vi "界面UI.vi"() -> ()   [LabVIEW 2016, in "超标留样集成.lvlib" / "德润DR803L超标留样.lvlib"]
uses:
  <vilib>/Utility/miscctls.llb/LVPointTypeDef.ctl
  <vilib>/Utility/config.llb/NI_LVConfig.lvlib
  <vilib>/ptbypt/NI_PtbyPt.lvlib
panel:
  out "流程计时/s":i32
  in  "单步控制":bool
  in  "设置":bool
  out "采样器进程 2":T1(ring)
  out "单次采样量":u16
  out "留样模式":T2(ring)
  out "门状态":enum16{"门开", "门关"}(ring)
  out "报警状态":enum16{"无报警", "缺水报警"}(ring)
  out "仪器时间":timestamp format="%<%Y/%m/%d %H:%M:%S>T"
  out "当前瓶号":u16
  out "采样器状态":enum16{"停止", "运行"}(ring)
  out "采样器进程":i32(listbox)
  out "流程中":bool
  in  "停止流程":bool
  in  "启动流程":bool
  in  "修改门禁密码":bool
  in  "远程复位":bool
  in  "远程留样":bool
  out "Registers":u16[](array[numeric])
  in  "采样启动":bool
  in  "停止命令":bool
  in  "切换采样器状态":bool
  in  "时间校准":bool
  out "通讯":bool
  # "只在待机时启动有效"
  # "德润DR803L超标留样"
  # "只在待机时启动有效"
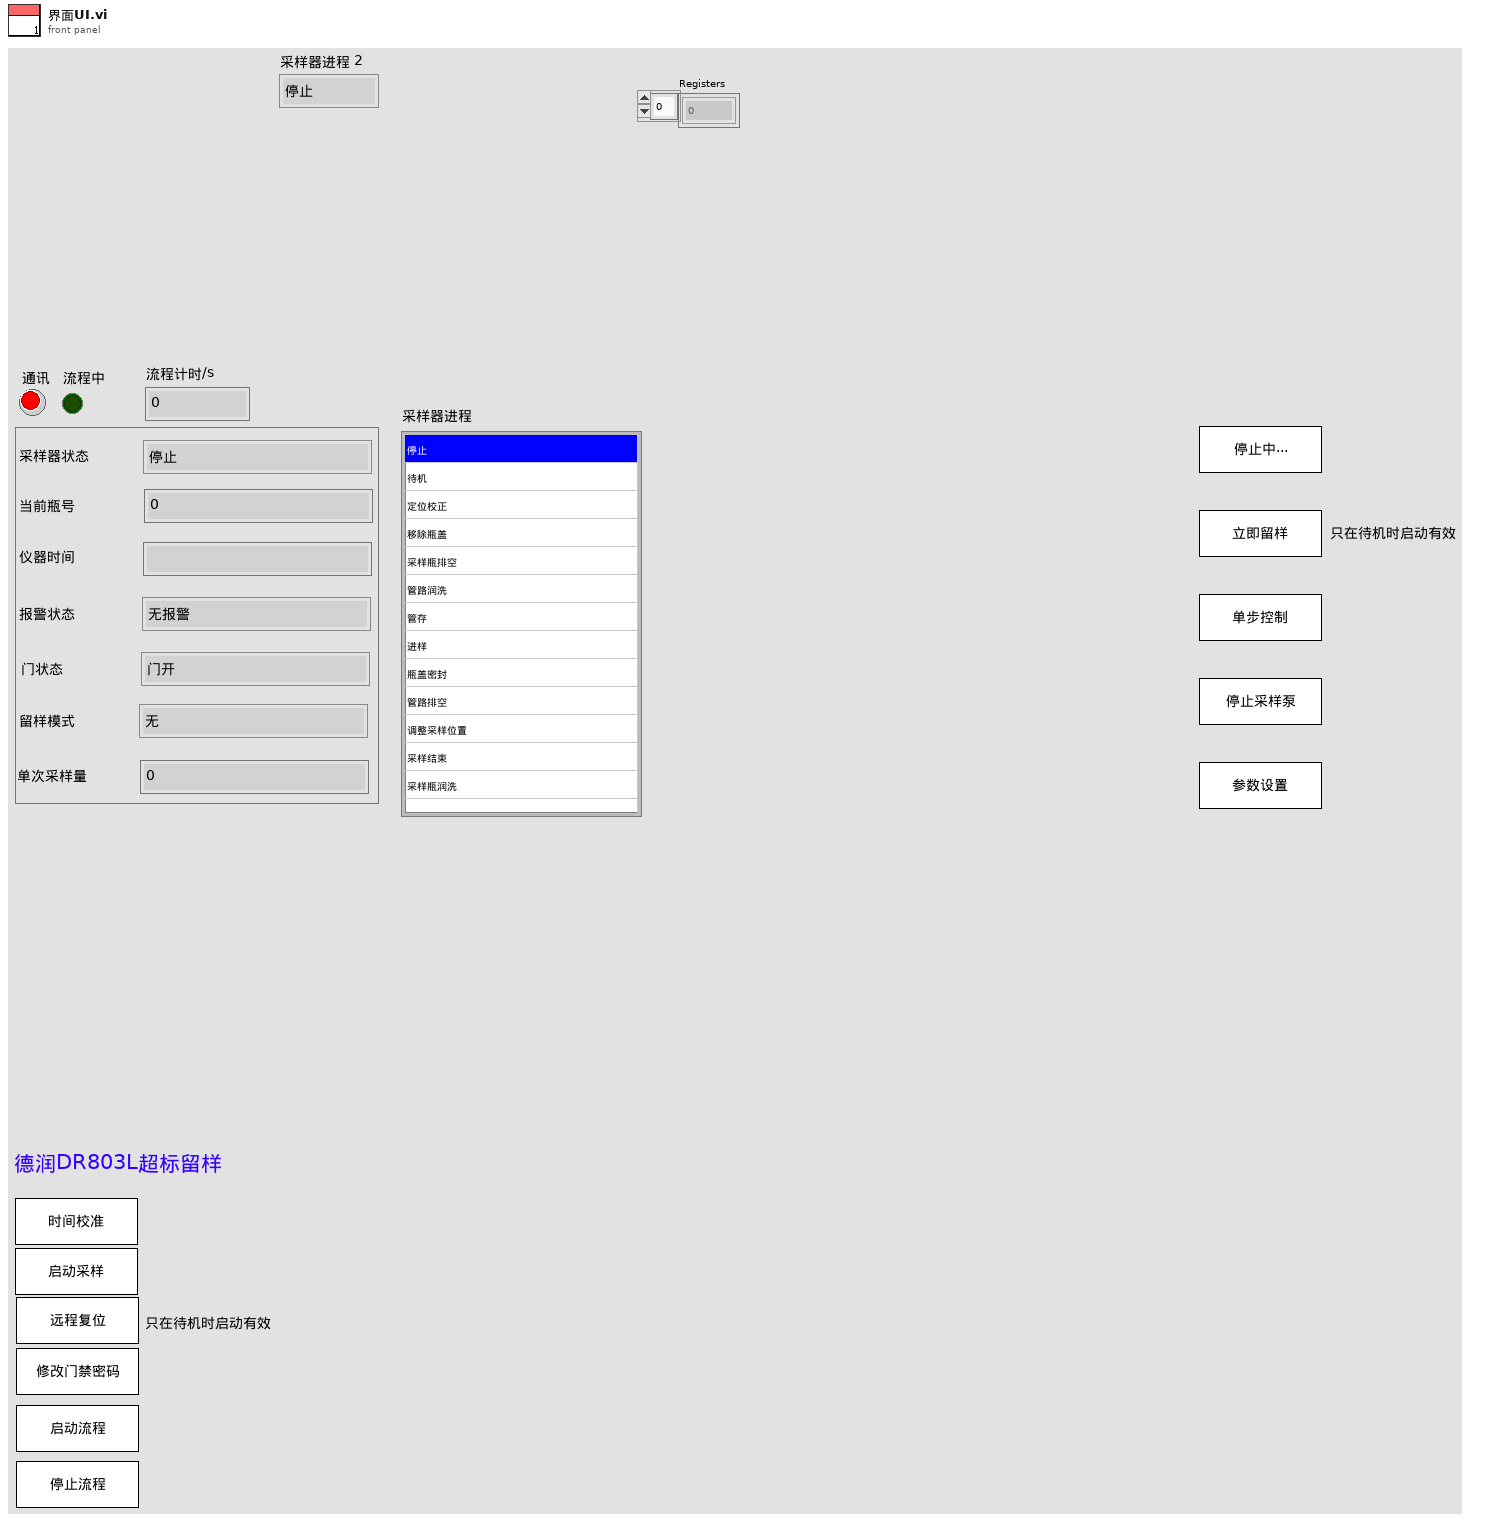
[diagram p1: front panel]
types:
  T1 = enum16{"停止", "待机", "定位校正", "移除瓶盖", "采样瓶排空", "管路润洗", "管存", "进样", "瓶盖密封", "管路排空", "调整采样位置", "采样结束", "采样瓶润洗", "瓶润洗排空"}
  T2 = enum16{"无", "定时留样", "时间等比例", "超标留样", "同步留样", "外控留样"}
  T3 = cluster{"STEP":enum16{"open", "read", "write", "write single", "close"}, "starting address":u16, "value":u16}
  T4 = typedef "LVPointTypeDef.ctl" = cluster{"Horizontal":i16, "Vertical":i16}
  T5 = typedef "NI_LVConfig.lvlib/Config Data RefNum.ctl" = refnum<k1>
  T6 = enum16{"open", "read", "write", "write single", "close"}
  T7 = typedef "LVDateTimeRec.ctl" = cluster{"秒数的小数部分":dbl, "秒":i32, "分":i32, "时":i32, "日":i32, "月":i32, "年":i32, "天数（周）":i32, "天数（年）":i32, "DST":i32}
  T8 = enum32{"Bad", "Idle", "Run top level", "Running"}
  T9 = cluster{"采样器状态":enum16{"停止", "运行"}, "当前留样瓶编号":u16, "报警状态":enum16{"无报警", "缺水报警"}, "超标信号":enum16{"无信号", "超标信号"}, "采样器进程":enum16{"停止", "待机", "定位校正", "移除瓶盖", "采样瓶排空", "管路润洗", "管存", "进样", "瓶盖密封", "管路排空", "调整采样位置", "采样结束", "采样瓶润洗", "瓶润洗排空"}, "版本号":string, "同步信号":enum16{"无信号", "同步信号"}, "外控信号":enum16{"无信号", "外控信号"}, "门状态":enum16{"门开", "门关"}, "当前瓶号":u16, "工作状态":enum16{"停止", "采样中"}, "留样模式":enum16{"无", "定时留样", "时间等比例", "超标留样", "同步留样", "外控留样"}, "立即留样":enum16{"无", "远程留样"}, "采样方式":enum16{"单采", "双重"}, "仪器时间":timestamp, "单次采样量":u16, "时间等比采样采样间隔":u16, "排空命令":u16, "远程复位":u16, "门禁密码":u16}
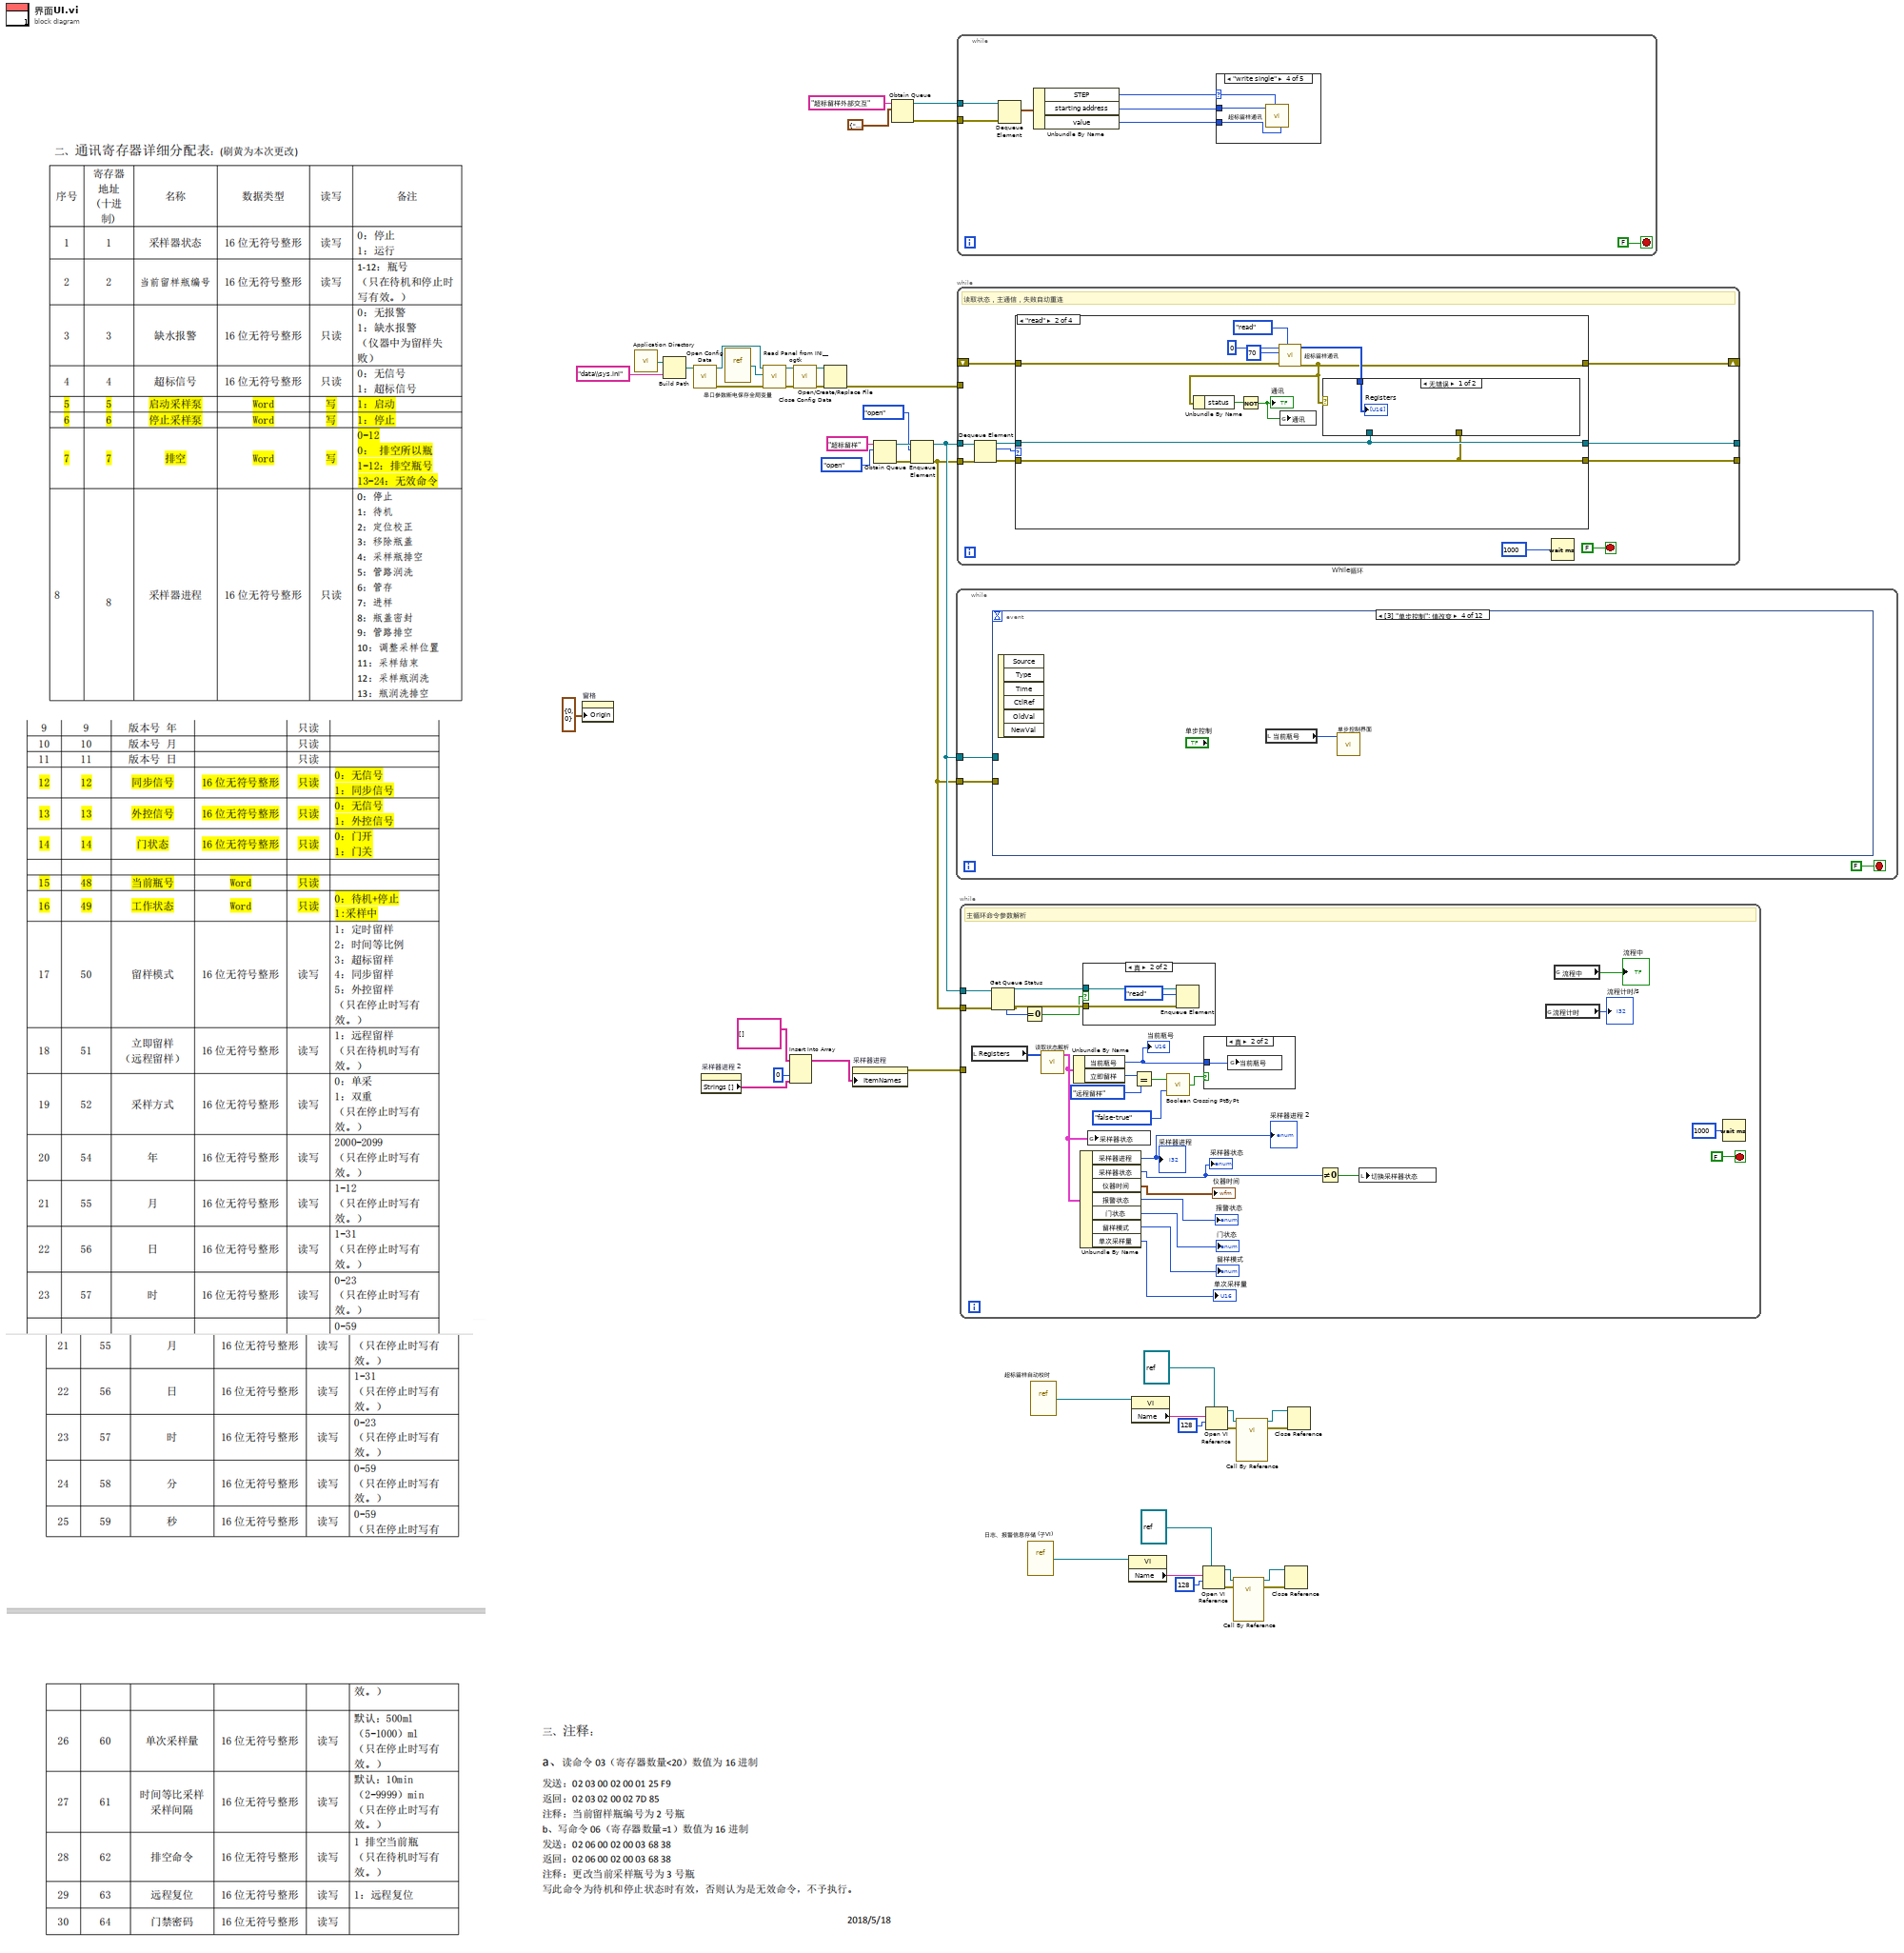
[diagram p0: block diagram]
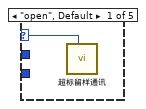
[diagram p2: hidden frame]
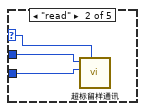
[diagram p3: hidden frame]
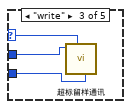
[diagram p4: hidden frame]
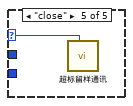
[diagram p5: hidden frame]
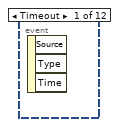
[diagram p6: hidden frame]
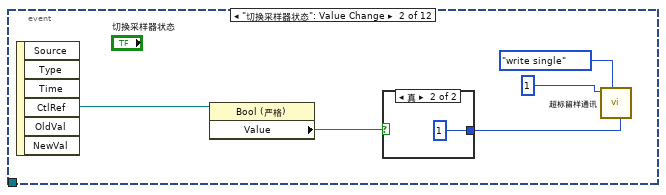
[diagram p7: hidden frame]
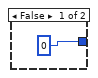
[diagram p8: hidden frame]
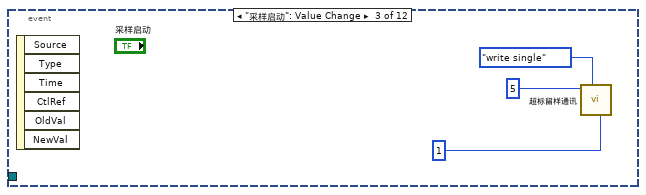
[diagram p9: hidden frame]
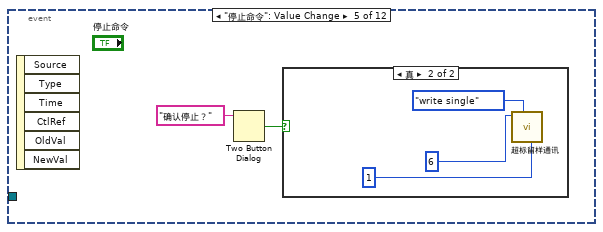
[diagram p10: hidden frame]
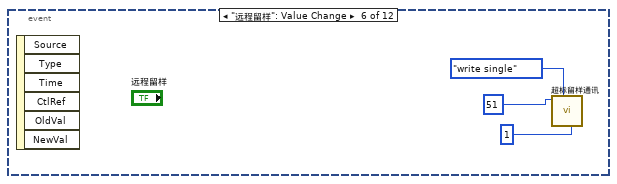
[diagram p12: hidden frame]
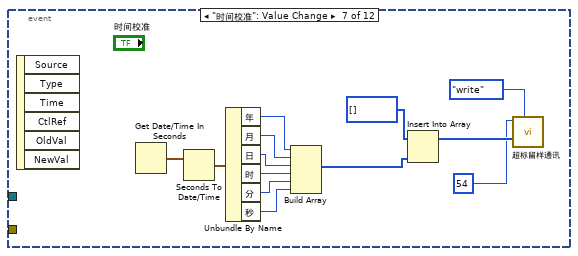
[diagram p13: hidden frame]
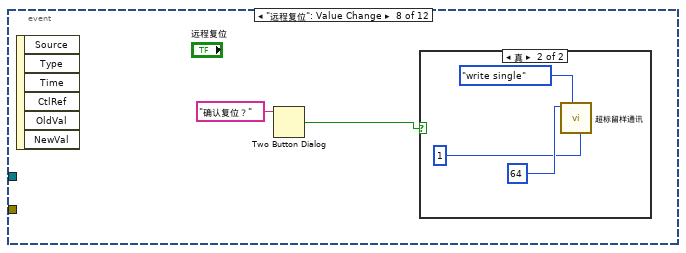
[diagram p14: hidden frame]
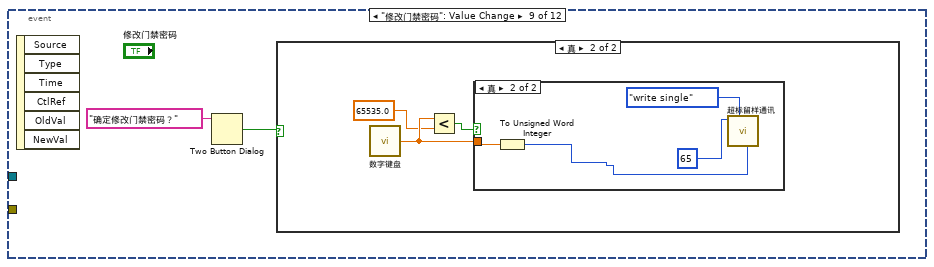
[diagram p16: hidden frame]
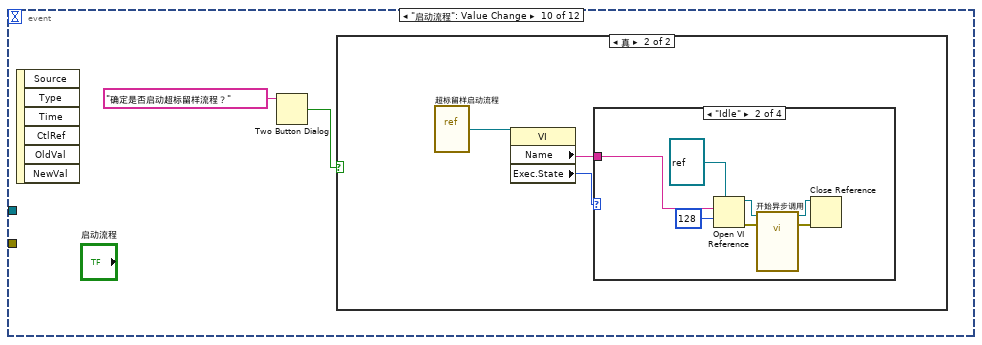
[diagram p19: hidden frame]
diagram:
  n1 = property on="窗格" class="Pane"("Origin"=T4 {"Horizontal"=0, "Vertical"=0} ("原点")) -> ()  [unwired: 2 in, 2 out]
  n2 = call <vilib>:"Application Directory.vi"() -> ("Application Directory"=w36:path)
  n3 = Build Path(base path=w36, name or relative path="data\\sys.ini" ("名称或相对路径")) -> (appended path=w34:path)
  n4 = call <vilib>:"Open Config Data.vi"("configuration file path"=w34) -> ("error out"=w30:errorcluster, "refnum"=w33:T5)  [unwired: 8 in, 1 out]
  n5 = property on="采样器进程 2" class="Enum (严格)"() -> ("Strings []"=w1:string[])  [unwired: 2 in, 2 out]
  n6 = vi-ref "串口参数断电保存全局变量.vi"() -> (w32:refnum<vi>)
  n7 = call <userlib>:"Read Panel from INI__ogtk.vi"("error in (no error)"=w30, "VI ref"=w32, "refnum"=w33) -> ("error out"=w29:errorcluster, "refnum out"=w31:T5)  [unwired: 7 in]
  n8 = Insert Into Array(array=string[][] [] ("字符串[]"), index (col)=0 ("禁用的索引 (列)"), new element=w1) -> (w3:string[][])  [unwired: 1 in]
  n9 = call <vilib>:"Close Config Data.vi"("error in (no error)"=w29, "refnum"=w31) -> ("error out"=w28:errorcluster, "file path"=w27:path)  [unwired: 8 in]
  n10 = Open/Create/Replace File(file path (use dialog)=w27, error in=w28) -> (error out=w26:errorcluster)  [unwired: 4 in, 2 out]
  n11 = property on="采样器进程" class="MCListbox (严格)"("ItemNames"=w3) -> (error out=w2:errorcluster)  [unwired: 2 in, 1 out]
  n12 = Obtain Queue(name (unnamed)="超标留样" ("名称（未命名）"), element data type=enum16{"open", "read", "write", "close"}."open") -> (queue out=w42:refnum<queue>, error out=w41:errorcluster)  [unwired: 3 in, 1 out]
  n13 = Obtain Queue(name (unnamed)="超标留样外部交互" ("名称（未命名）"), element data type=T3 {"STEP"=enum."write single", "starting address"=0, "value"=0}) -> (queue out=w23:refnum<queue>, error out=w22:errorcluster)  [unwired: 3 in, 1 out]
  n14 = Enqueue Element(queue=w42, element=enum16{"open", "read", "write", "close"}."open", error in (no error)=w41) -> (queue out=w39:refnum<queue>, error out=w38:errorcluster)  [unwired: 1 in, 1 out]
  n15 = while {
    tunnel: w39 -> [w46]
    tunnel: w38 -> [w45]
    stop <- FALSE stop-if-true
    n16 = event shown="[3] \"单步控制\": 值改变" {
      selector: _ -> [_ _ _ _ _ _ _ _ _ _ _ _]
      dyn-events: _ -> [_ _ _ _ _ _ _ _ _ _ _ _]
      timeout: _ -> [_ _ _ _ _ _ _ _ _ _ _ _]
      tunnel: w46 -> [_ _ _ _ _ _ _ _ _ _ _ _]
      tunnel: w45 -> [_ _ _ _ _ _ _ _ _ _ _ _]
      event Timeout {
        n17 = event-data() -> ()  [unwired: 1 in, 3 out]
      }
      event "切换采样器状态": Value Change {
        n18 = event-data() -> ("CtlRef"=w52:refnum<vi>)  [unwired: 1 in, 5 out]
        n19 = property class="Bool (严格)"(reference=w52) -> ("Value"=w51:bool)  [unwired: 1 in, 2 out]
        n20 = case shown="真" w51 {
          tunnel: [u16 0 ("索引") u16 1 ("索引")] -> w48
          frame False {
          }
          frame True {
          }
        }
        n21 = call "超标留样通讯.vi"("value"=w48, "STEP"=T6."write single", "starting address"=1 ("索引")) -> ()  [unwired: 6 in, 3 out]
      }
      event "采样启动": Value Change {
        n22 = event-data() -> ()  [unwired: 1 in, 6 out]
        n23 = call "超标留样通讯.vi"("value"=u16 1 ("新元素/子数组"), "STEP"=T6."write single", "starting address"=5 ("索引")) -> ()  [unwired: 6 in, 3 out]
      }
      event "单步控制": Value Change {
        n24 = event-data() -> ()  [unwired: 1 in, 6 out]
        n25 = local read "当前瓶号"() -> (w58:u16)
        n26 = call "单步控制界面.vi"("当前瓶号"=w58) -> ()  [unwired: 11 in]
      }
      event "停止命令": Value Change {
        n27 = event-data() -> ()  [unwired: 1 in, 6 out]
        n28 = Two Button Dialog(message="确认停止？" ("消息")) -> (T button?=w59:bool)  [unwired: 2 in]
        n29 = case shown="真" w59 {
          frame False {
          }
          frame True {
            n30 = call "超标留样通讯.vi"("value"=u16 1 ("新元素/子数组"), "STEP"=T6."write single", "starting address"=6 ("索引")) -> ()  [unwired: 6 in, 3 out]
          }
        }
      }
      event "远程留样": Value Change {
        n31 = event-data() -> ()  [unwired: 1 in, 6 out]
        n32 = call "超标留样通讯.vi"("value"=u16 1 ("新元素/子数组"), "STEP"=T6."write single", "starting address"=51 ("索引")) -> ()  [unwired: 6 in, 3 out]
      }
      event "时间校准": Value Change {
        n33 = event-data() -> ()  [unwired: 1 in, 6 out]
        n34 = Get Date/Time In Seconds() -> (seconds since 1Jan1904=w79:timestamp)
        n35 = Seconds To Date/Time(time stamp (now)=w79) -> (date time rec=w78:T7)  [unwired: 1 in]
        n36 = Unbundle By Name(w78) -> ("年"=w75:i32, "月"=w74:i32, "日"=w73:i32, "时"=w72:i32, "分"=w71:i32, "秒"=w70:i32)
        n37 = Build Array(w75, w74, w73, w72, w71, w70) -> (w69:i32[])
        n38 = Insert Into Array(array=u16[] [] ("values"), new element=w69) -> (w76:u16[])  [unwired: 1 in]
        n39 = call "超标留样通讯.vi"("STEP"=T6."write", "values"=w76, "starting address"=54 ("索引")) -> ()  [unwired: 6 in, 3 out]
      }
      event "远程复位": Value Change {
        n40 = event-data() -> ()  [unwired: 1 in, 6 out]
        n41 = Two Button Dialog(message="确认复位？" ("消息")) -> (T button?=w80:bool)  [unwired: 2 in]
        n42 = case shown="真" w80 {
          frame False {
          }
          frame True {
            n43 = call "超标留样通讯.vi"("value"=u16 1 ("新元素/子数组"), "STEP"=T6."write single", "starting address"=64 ("索引")) -> ()  [unwired: 6 in, 3 out]
          }
        }
      }
      event "修改门禁密码": Value Change {
        n44 = event-data() -> ()  [unwired: 1 in, 6 out]
        n45 = Two Button Dialog(message="确定修改门禁密码？" ("消息")) -> (T button?=w85:bool)  [unwired: 2 in]
        n46 = case shown="真" w85 {
          frame False {
          }
          frame True {
            n47 = call "数字键盘.vi"() -> ("NewNumber"=w89:sgl)  [unwired: 1 in]
            n48 = Less?(x=w89, y=sgl 65535.0) -> (x < y?=w87:bool)
            n49 = case shown="真" w87 {
              tunnel: w89 -> [_ w93]
              frame False {
              }
              frame True {
                n50 = To Unsigned Word Integer(number=w93) -> (unsigned 16bit integer=w90:u16)
                n51 = call "超标留样通讯.vi"("value"=w90, "STEP"=T6."write single", "starting address"=65 ("索引")) -> ()  [unwired: 6 in, 3 out]
              }
            }
          }
        }
      }
      event "启动流程": Value Change {
        n52 = event-data() -> ()  [unwired: 1 in, 6 out]
        n53 = Two Button Dialog(message="确定是否启动超标留样流程？" ("消息")) -> (T button?=w94:bool)  [unwired: 2 in]
        n54 = case shown="真" w94 {
          frame False {
          }
          frame True {
            n55 = vi-ref "超标留样启动流程.vi"() -> (w96:refnum<vi>)
            n56 = property class="VI"(reference=w96) -> ("Name"=w97:string, "Exec.State"=w98:T8)  [unwired: 1 in, 2 out]
            n57 = case shown="\"Idle\"" w98 {
              tunnel: w97 -> [_ w101 _ _]
              frame "Bad", Default {
              }
              frame "Idle" {
                n58 = Open VI Reference(type specifier VI Refnum (for type only)=refnum<vi> refnum ("类型说明符VI引用句柄（仅用于类型）"), vi path=w101, options=128 ("选项")) -> (vi reference=w105:refnum<vi>, error out=w100:errorcluster)  [unwired: 3 in]
                n59 = call-by-ref "开始异步调用"(reference=w105, error in=w100) -> (reference out=w104:refnum<vi>, error out=w99:errorcluster)  [unwired: 12 in]
                n60 = Close Reference(reference=w104, error in (no error)=w99) -> ()  [unwired: 1 out]
              }
              frame "Run top level" {
              }
              frame "Running" {
              }
            }
          }
        }
      }
      event "停止流程": Value Change {
        n61 = event-data() -> ()  [unwired: 1 in, 6 out]
        n62 = Two Button Dialog(message="确定是否停止超标留样流程并排空当前瓶？" ("消息")) -> (T button?=w106:bool)  [unwired: 2 in]
        n63 = case shown="真" w106 {
          frame False {
          }
          frame True {
            n64 = Obtain Notifier(name (unnamed)="超标留样流程" ("名称（未命名）"), notification data type=FALSE ("采样完成")) -> (notifier out=w119:refnum<notifier>, error out=w118:errorcluster)  [unwired: 2 in, 1 out]
            n65 = Send Notification(notification=TRUE ("通知"), notifier=w119, error in (no error)=w118) -> (notifier out=w116:refnum<notifier>, error out=w115:errorcluster)
            n66 = call "超标留样通讯.vi"("value"=u16 1 ("新元素/子数组"), "STEP"=T6."write single", "starting address"=6 ("索引")) -> ("error out"=w108:errorcluster)  [unwired: 6 in, 2 out]
            n67 = Release Notifier(notifier=w116, error in (no error)=w115) -> ()  [unwired: 1 in, 3 out]
            n68 = call "超标留样通讯.vi"("value"=u16 1 ("新元素/子数组"), "STEP"=T6."write single", "Error in"=w108, "starting address"=63 ("索引")) -> ()  [unwired: 5 in, 3 out]
          }
        }
      }
      event "设置": Value Change {
        n69 = event-data() -> ()  [unwired: 1 in, 6 out]
        n70 = global read "超标留样全局.vi" "采样器状态"() -> (w126:T9)
        n71 = Unbundle By Name(w126) -> ("留样模式"=w125:T2, "采样方式"=w124:enum16{"单采", "双重"}, "单次采样量"=w123:u16, "时间等比采样采样间隔"=w122:u16)
        n72 = call "参数设置对画框.vi"("时间等比采样"=w122, "单次采样量"=w123, "采样方式"=w124, "留样模式"=w125) -> ()  [unwired: 8 in]
      }
    }
  }
  n73 = while {
    tunnel: w23 -> [w132]
    tunnel: w22 -> [w131]
    stop <- FALSE stop-if-true
    n74 = Dequeue Element(queue=w132, error in (no error)=w131) -> (element=w130:T3)  [unwired: 1 in, 3 out]
    n75 = Unbundle By Name(w130) -> ("STEP"=w129:T6, "starting address"=w128:u16, "value"=w127:u16)
    n76 = case shown="\"write single\"" w129 {
      selector: w129 -> [w134 w137 w140 w143 w144]
      tunnel: w128 -> [_ w136 w139 w142 _]
      tunnel: w127 -> [_ w135 w138 w141 _]
      frame "open", Default {
        n77 = call "超标留样通讯.vi"("STEP"=w134) -> ()  [unwired: 8 in, 3 out]
      }
      frame "read" {
        n78 = call "超标留样通讯.vi"("STEP"=w137, "quantity"=w135, "starting address"=w136) -> ()  [unwired: 6 in, 3 out]
      }
      frame "write" {
        n79 = call "超标留样通讯.vi"("value"=w138, "STEP"=w140, "starting address"=w139) -> ()  [unwired: 6 in, 3 out]
      }
      frame "write single" {
        n80 = call "超标留样通讯.vi"("value"=w141, "STEP"=w143, "starting address"=w142) -> ()  [unwired: 6 in, 3 out]
      }
      frame "close" {
        n81 = call "超标留样通讯.vi"("STEP"=w144) -> ()  [unwired: 8 in, 3 out]
      }
    }
  }
  n82 = while "While循环" {
    tunnel: w39 -> [w146]
    tunnel: w38 -> [w145]
    tunnel: [w150] -> _
    tunnel: [w149] -> _
    shift-right: [w147] -> _
    shift-left: _ -> [w148]
    tunnel: w26 -> [_]
    stop <- FALSE stop-if-true
    # "读取状态，主通信，失败自动重连"
    n83 = Dequeue Element(queue=w146, error in (no error)=w145) -> (queue out=w152:refnum<queue>, element=w153:enum16{"open", "read", "write", "close"}, error out=w151:errorcluster)  [unwired: 1 in, 1 out]
    n84 = case shown="\"read\"" w153 {
      tunnel: [w161 w163 w181 w190] -> w147
      tunnel: w152 -> [w160 w166 w180 w193]
      tunnel: w151 -> [w159 w165 w179 w192]
      tunnel: [w160 w166 w180 w193] -> w150
      tunnel: [w159 w165 w179 w192] -> w149
      tunnel: w148 -> [w158 w171 w183 w194]
      frame "open", Default {
        n85 = call "超标留样通讯.vi"("STEP"=T6."open", "Error in"=w158) -> ("error out"=w161:errorcluster, "MB session in"=w157:refnum<class "MB_Master.lvclass">)  [unwired: 7 in, 1 out]
        n86 = global write "串口参数断电保存全局变量.vi" "MB session in"(w157) -> ()
      }
      frame "read" {
        n87 = call "超标留样通讯.vi"("STEP"=T6."read", "Error in"=w171, "quantity"=u16 70, "starting address"=u16 0) -> ("error out"=w163:errorcluster, "Registers"=w168:u16[])  [unwired: 5 in, 1 out]
        n88 = Unbundle By Name(w163) -> ("status"=w164:bool)
        n89 = Not(x=w164) -> (.not. x?=w162:bool)
        "通讯" <- w162
        n90 = global write "超标留样全局.vi" "通讯"(w162) -> ()
        n91 = case shown="无错误" w163 {
          tunnel: w168 -> [w172 _]
          tunnel: w166 -> [_ w177]
          tunnel: w165 -> [_ w176]
          frame No Error {
            "Registers" <- w172
          }
          frame Error {
            n92 = Enqueue Element(queue=w177, element=enum16{"open", "read", "write", "close"}."close" ("元素"), error in (no error)=w176) -> (queue out=w175:refnum<queue>, error out=w174:errorcluster)  [unwired: 1 in, 1 out]
            n93 = Enqueue Element(queue=w175, element=enum16{"open", "read", "write", "close"}."open" ("元素"), error in (no error)=w174) -> ()  [unwired: 1 in, 3 out]
          }
        }
      }
      frame "write" {
        n94 = call "超标留样通讯.vi"("STEP"=T6."write single", "Error in"=w183) -> ("error out"=w181:errorcluster)  [unwired: 7 in, 2 out]
        n95 = case shown="错误" w181 {
          tunnel: w180 -> [_ w185]
          tunnel: w179 -> [_ w184]
          frame No Error {
          }
          frame Error {
            n96 = Enqueue Element(queue=w185, element=enum16{"open", "read", "write", "close"}."close" ("元素"), error in (no error)=w184) -> (queue out=w188:refnum<queue>, error out=w187:errorcluster)  [unwired: 1 in, 1 out]
            n97 = Enqueue Element(queue=w188, element=enum16{"open", "read", "write", "close"}."open" ("元素"), error in (no error)=w187) -> ()  [unwired: 1 in, 3 out]
          }
        }
      }
      frame "close" {
        n98 = call "超标留样通讯.vi"("STEP"=T6."close", "Error in"=w194) -> ("error out"=w190:errorcluster)  [unwired: 7 in, 2 out]
      }
    }
    n99 = Wait (ms)(milliseconds to wait=u32 1000 ("等待时间（毫秒）")) -> ()  [unwired: 1 out]
  }
  n100 = while {
    tunnel: w39 -> [w218]
    tunnel: w38 -> [w217]
    tunnel: w2 -> [_]
    stop <- FALSE stop-if-true
    # "主循环命令参数解析"
    n101 = local read "Registers"() -> (w212:u16[])
    n102 = Get Queue Status(queue=w218, error in (no error)=w217) -> (queue out=w215:refnum<queue>, error out=w214:errorcluster, # elements in queue=w216:i32)  [unwired: 1 in, 5 out]
    n103 = Equal To 0?(x=w216) -> (x = 0?=w213:bool)
    n104 = call "读取状态解析.vi"("Registers"=w212) -> ("采样器状态"=w205:T9)  [unwired: 9 in, 1 out]
    n105 = Unbundle By Name(w205) -> ("当前瓶号"=w204:u16, "立即留样"=w211:enum16{"无", "远程留样"})
    "当前瓶号" <- w204
    n106 = Unbundle By Name(w205) -> ("采样器进程"=→"采样器进程" →"采样器进程 2":T1, "采样器状态"=w197:enum16{"停止", "运行"}, "仪器时间"=→"仪器时间":timestamp, "报警状态"=→"报警状态":enum16{"无报警", "缺水报警"}, "门状态"=→"门状态":enum16{"门开", "门关"}, "留样模式"=→"留样模式":T2, "单次采样量"=→"单次采样量":u16)
    "采样器状态" <- w197
    n107 = case shown="真" w213 {
      tunnel: w215 -> [_ w223]
      tunnel: w214 -> [_ w222]
      frame False {
      }
      frame True {
        n108 = Enqueue Element(queue=w223, element=enum16{"open", "read", "write", "close"}."read" ("元素"), error in (no error)=w222) -> ()  [unwired: 1 in, 3 out]
      }
    }
    n109 = global write "超标留样全局.vi" "采样器状态"(w205) -> ()
    n110 = Equal?(x=w211, y=enum16{"无", "远程留样"}."远程留样") -> (x = y?=w210:bool)
    n111 = call <vilib>:"Boolean Crossing PtByPt.vi"("direction"=enum16{"either", "false-true", "true-false"}."false-true", "input"=w210) -> ("crossing"=w208:bool)  [unwired: 1 in]
    n112 = case shown="真" w208 {
      tunnel: w204 -> [_ w221]
      frame False {
      }
      frame True {
        n113 = global write "超标留样全局.vi" "当前瓶号"(w221) -> ()
      }
    }
    n114 = Not Equal To 0?(x=w197) -> (x != 0?=w196:bool)
    n115 = local write "切换采样器状态"(w196) -> ()
    n116 = global read "串口参数断电保存全局变量.vi" "流程计时"() -> (→"流程计时/s":i32)
    n117 = global read "串口参数断电保存全局变量.vi" "流程中"() -> (→"流程中":bool)
    n118 = Wait (ms)(milliseconds to wait=u32 1000 ("等待时间（毫秒）")) -> ()  [unwired: 1 out]
  }
  n119 = vi-ref "日志、报警信息存储 (子VI).vi"() -> (w14:refnum<vi>)
  n120 = vi-ref "超标留样自动校时.vi"() -> (w13:refnum<vi>)
  n121 = property class="VI"(reference=w14) -> ("Name"=w15:string)  [unwired: 1 in, 2 out]
  n122 = property class="VI"(reference=w13) -> ("Name"=w12:string)  [unwired: 1 in, 2 out]
  n123 = Open VI Reference(type specifier VI Refnum (for type only)=refnum<vi> refnum, vi path=w15, options=128 ("选项")) -> (vi reference=w17:refnum<vi>, error out=w19:errorcluster)  [unwired: 3 in]
  n124 = Open VI Reference(type specifier VI Refnum (for type only)=refnum<vi> refnum, vi path=w12, options=128 ("选项")) -> (vi reference=w10:refnum<vi>, error out=w8:errorcluster)  [unwired: 3 in]
  n125 = call-by-ref "?"(reference=w17, error in=w19) -> (reference out=w21:refnum<vi>, error out=w20:errorcluster)  [unwired: 12 in]
  n126 = call-by-ref "?"(reference=w10, error in=w8) -> (reference out=w6:refnum<vi>, error out=w7:errorcluster)  [unwired: 12 in]
  n127 = Close Reference(reference=w21, error in (no error)=w20) -> ()  [unwired: 1 out]
  n128 = Close Reference(reference=w6, error in (no error)=w7) -> ()  [unwired: 1 out]
